vi "动态调用.vi"(10 "VI路径":path) -> ()   [LabVIEW 2018]
panel:
  out "错误输出":errorcluster
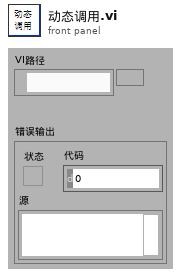
[diagram p1: front panel]
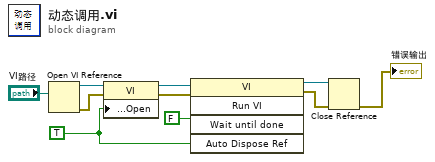
[diagram p0: block diagram]
diagram:
  w5 = TRUE ("结束前等待")
  n1 = Open VI Reference(vi path="VI路径") -> (vi reference=w10:refnum<vi>, error out=w7:errorcluster)  [unwired: 5 in]
  n2 = property on="Property Node" class="VI"(reference=w10, error in=w7, "Front Panel Window:Open"=w5) -> (reference out=w9:refnum<vi>, error out=w8:errorcluster)
  n3 = invoke class="VI" method="Run VI"(reference=w9, error in=w8, "Wait until done"=FALSE ("结束前等待"), "Auto Dispose Ref"=w5) -> (reference out=w4:refnum<vi>, error out=w3:errorcluster)  [unwired: 1 in, 3 out]
  n4 = Close Reference(reference=w4, error in (no error)=w3) -> (error out=→"错误输出":errorcluster)
